vi "mm to points.vi"(3 "mm":sgl) -> (0 "points":sgl)   [LabVIEW 2013]
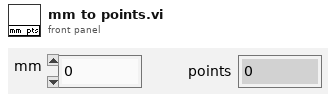
[diagram p1: front panel]
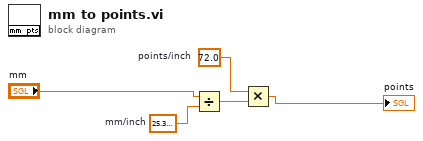
[diagram p0: block diagram]
diagram:
  w3 = sgl 25.4  # mm/inch
  w4 = sgl 72.0  # points/inch
  n1 = Divide(x="mm", y=w3) -> (x/y=w5:sgl)
  n2 = Multiply(x=w4, y=w5) -> (x*y=→"points":sgl)
